vi "Unflatten From MessagePack.vi"(8 "error in (no error)":errorcluster, 11 "MsgPack Data":string) -> (0 "error IO":errorcluster, 3 "Data":variant)   [LabVIEW 2015, in "MsgPackDeserializer.lvclass"]
uses:
  MsgPackDeserializer.lvclass
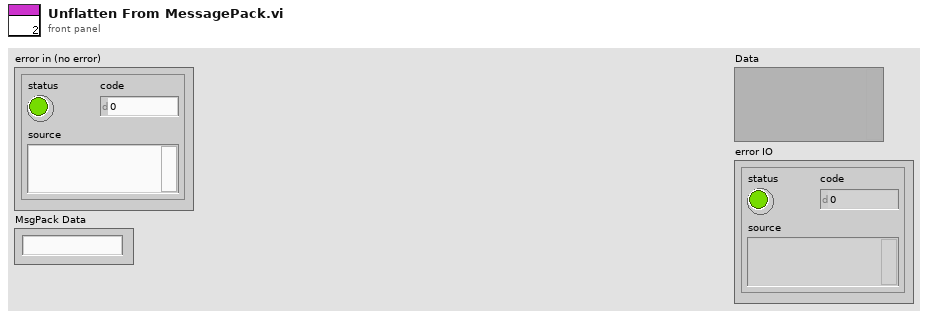
[diagram p1: front panel]
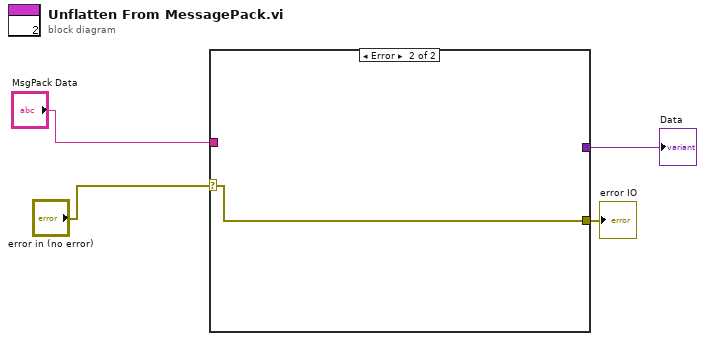
[diagram p0: block diagram]
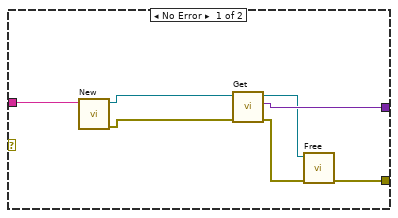
[diagram p2: hidden frame]
diagram:
  n1 = case shown="Error" "error in (no error)" {
    selector: "error in (no error)" -> [_ w12]
    tunnel: "MsgPack Data" -> [w9 _]
    tunnel: [w8 _] -> w2
    tunnel: [w5 w12] -> w1
    frame No Error {
      n2 = call "New.vi"("MsgPack Data"=w9) -> ("error out"=w10:errorcluster, "Deserializer"=w11:refnum<class "MsgPackDeserializer.lvclass">)  [unwired: 9 in]
      n3 = call "Get.vi"("error in (no error)"=w10, "MsgPackDeserializer in"=w11) -> ("error out"=w6:errorcluster, "Variant"=w8:variant, "MsgPackDeserializer out"=w7:refnum<class "MsgPackDeserializer.lvclass">)  [unwired: 7 in]
      n4 = call "Free.vi"("error in (no error)"=w6, "MsgPackDeserializer.lvclass"=w7) -> ("error IO"=w5:errorcluster)  [unwired: 8 in, 1 out]
    }
    frame Error {
    }
  }
  "Data" <- w2
  "error IO" <- w1
